vi "Optimizer.vi"() -> ()   [LabVIEW 2018]
panel:
  in  "Optimizer":enum16{"Adagrad", "Adadelta", "Adam"}(ring)
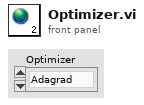
[diagram p1: front panel]
diagram:
